vi "Start sshd.vi"(8 "error in (no error)":errorcluster, 10 "arguments":string) -> (0 "error out":errorcluster, 3 "Process":refnum<k24>)   [LabVIEW 2013, in "libssh2_integration_tests.lvlib" / "Server Fixture.lvclass"]
doc: "Execute sshd as process (\"-D\") with specified arguments."
uses:
  Server Fixture.lvclass
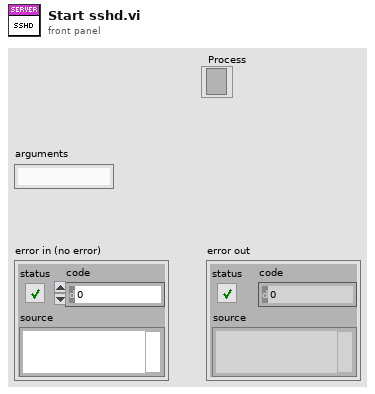
[diagram p1: front panel]
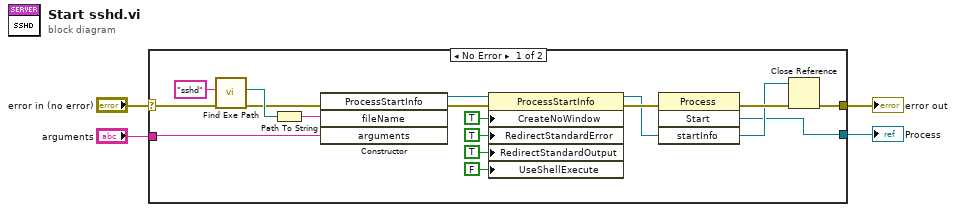
[diagram p0: block diagram]
diagram:
  n1 = case shown="No Error" "error in (no error)" {
    selector: "error in (no error)" -> [w21 w22]
    tunnel: "arguments" -> [w6 _]
    tunnel: [w11 w22] -> w3
    tunnel: [w10 _] -> w1
    frame No Error {
      n2 = call "Find Exe Path.vi"("error in (no error)"=w21, "executable"="sshd") -> ("error out"=w5:errorcluster, "path"=w7:path)  [unwired: 8 in]
      n3 = Path To String(path=w7) -> (string=w8:string)
      n4 = constructor class="ProcessStartInfo"(error in=w5, "fileName"=w8, "arguments"=w6) -> (reference out=w18:refnum<k24>, error out=w20:errorcluster)  [unwired: 2 in, 3 out]
      n5 = property class="ProcessStartInfo"(reference=w18, error in=w20, "CreateNoWindow"=TRUE, "RedirectStandardError"=TRUE, "RedirectStandardOutput"=TRUE, "UseShellExecute"=FALSE) -> (reference out=w12:refnum<k24>, error out=w19:errorcluster)
      n6 = invoke class="Process" method="Start"(error in=w19, "startInfo"=w12) -> (error out=w13:errorcluster, "Start"=w10:refnum<k24>)  [unwired: 2 in, 2 out]
      n7 = Close Reference(reference=w12, error in (no error)=w13) -> (error out=w11:errorcluster)
    }
    frame Error {
    }
  }
  "error out" <- w3
  "Process" <- w1
